vi "timestamp_string.vi"(3 "make file friendly":bool) -> (1 "timestamp string":string)   [LabVIEW 2024]
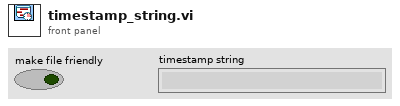
[diagram p1: front panel]
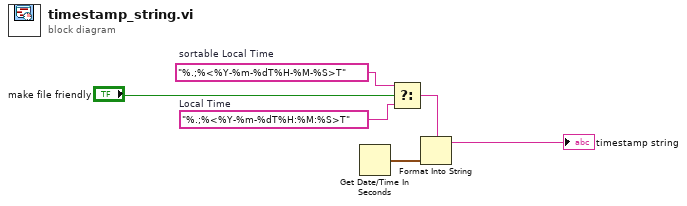
[diagram p0: block diagram]
diagram:
  w4 = "%.;%<%Y-%m-%dT%H-%M-%S>T"  # sortable Local Time
  w3 = "%.;%<%Y-%m-%dT%H:%M:%S>T"  # Local Time
  n1 = Get Date/Time In Seconds() -> (seconds since 1Jan1904=w6:timestamp)
  n2 = Select(t=w4, s="make file friendly", f=w3) -> (s? t:f=w1:string)
  n3 = Format Into String(format string=w1, w6) -> (resulting string=→"timestamp string":string)  [unwired: 2 in, 1 out]
